vi "Test Write Numerics.vi"(11 "TwinCAT ADS in":refnum<class "TwinCAT ADS.lvclass">) -> (3 "TwinCAT ADS out":refnum<class "TwinCAT ADS.lvclass">)   [LabVIEW 2018]
uses:
  TwinCAT ADS Class/TwinCAT ADS.lvclass
  e70a270d-43c8-4a10-98cb-cdcae2374215.vi
  06e0a99b-7b81-4ca8-a89e-7945807debb3.vi
  d8425a7c-cb21-4544-a4a3-9ee7345751d4.vi
  60045c97-3d21-4f52-bb28-386babca6960.vi
  96827efc-f82d-4e1c-9c1b-454960b395ec.vi
  7e66dc0a-1568-47cd-9851-5dc7b9fa6012.vi
  58f04dc6-9466-4392-88d8-370a7d168ec8.vi
  7dc634db-efdd-42f4-a4b0-d96c414e946f.vi
  TwinCAT ADS Class/VIs/Data/Read.vi
  <vilib>/addons/_JKI Toolkits/Caraya/classes/Assert/Assert Equal Value and Type_Variant.vi
  <vilib>/addons/_JKI Toolkits/Caraya/classes/Assert/Assert Almost Equal_Float.vi
  <vilib>/addons/_JKI Toolkits/Caraya/classes/Assert/Assert.lvclass
  <vilib>/addons/_JKI Toolkits/Caraya/classes/Test/Test.lvclass
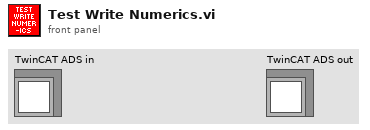
[diagram p1: front panel]
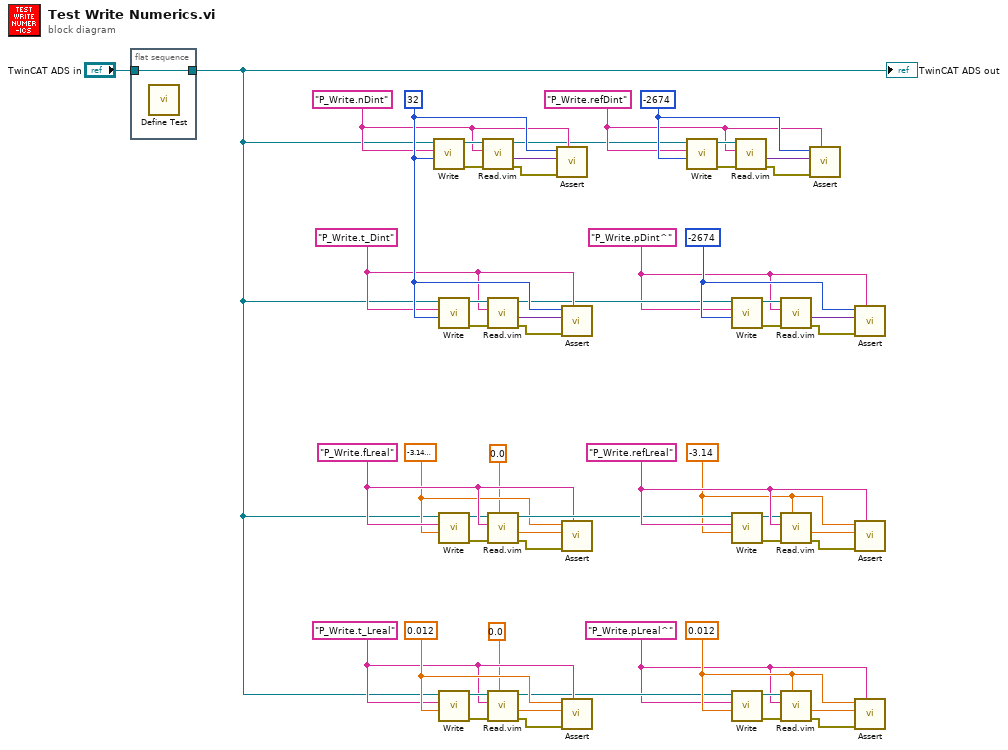
[diagram p0: block diagram]
diagram:
  w14 = 0.012
  w16 = 0.012 ("Value")
  w4 = "P_Write.pLreal^" ("Symbol Name")
  w10 = "P_Write.t_Lreal" ("Symbol Name")
  w19 = -3.140000104904175
  w17 = -3.14 ("Value")
  w29 = "P_Write.refLreal" ("Symbol Name")
  w23 = "P_Write.fLreal" ("Symbol Name")
  w32 = -2674 ("Value")
  w30 = "P_Write.pDint^" ("Symbol Name")
  w39 = -2674 ("Value")
  w38 = "P_Write.refDint" ("Symbol Name")
  w44 = "P_Write.t_Dint" ("Symbol Name")
  w46 = 32 ("Value")
  w45 = "P_Write.nDint" ("Symbol Name")
  n1 = flat-sequence {
    tunnel: "TwinCAT ADS in" -> [w56]
    tunnel: [w56] -> w3
    frame #0 {
      n2 = call <vilib>:"Define Test.vi"() -> ()  [unwired: 10 in, 2 out]
    }
  }
  n3 = call "Write.vi"("Value"=w46, "Symbol Name"=w45, "TwinCAT ADS in"=w3) -> ("error out"=w53:errorcluster, "TwinCAT ADS out"=w54:refnum<class "TwinCAT ADS.lvclass">)  [unwired: 7 in]
  n4 = call "Write.vi"("Value"=w46, "Symbol Name"=w44, "TwinCAT ADS in"=w3) -> ("error out"=w48:errorcluster, "TwinCAT ADS out"=w47:refnum<class "TwinCAT ADS.lvclass">)  [unwired: 7 in]
  n5 = call "Write.vi"("Value"=w19, "Symbol Name"=w23, "TwinCAT ADS in"=w3) -> ("error out"=w21:errorcluster, "TwinCAT ADS out"=w22:refnum<class "TwinCAT ADS.lvclass">)  [unwired: 7 in]
  n6 = call "Write.vi"("Value"=w14, "Symbol Name"=w10, "TwinCAT ADS in"=w3) -> ("error out"=w12:errorcluster, "TwinCAT ADS out"=w11:refnum<class "TwinCAT ADS.lvclass">)  [unwired: 7 in]
  n7 = call "Read.vim"("error in (no error)"=w53, "Symbol Name"=w45, "TwinCAT ADS in"=w54) -> ("error out"=w52:errorcluster, "Value"=w51:variant, "TwinCAT ADS out"=w37:refnum<class "TwinCAT ADS.lvclass">)  [unwired: 6 in]
  n8 = call "Read.vim"("error in (no error)"=w48, "Symbol Name"=w44, "TwinCAT ADS in"=w47) -> ("error out"=w49:errorcluster, "Value"=w50:variant, "TwinCAT ADS out"=w31:refnum<class "TwinCAT ADS.lvclass">)  [unwired: 6 in]
  n9 = call "Read.vim"("Type"=0.0, "error in (no error)"=w21, "Symbol Name"=w23, "TwinCAT ADS in"=w22) -> ("error out"=w20:errorcluster, "Value"=w18:dbl, "TwinCAT ADS out"=w28:refnum<class "TwinCAT ADS.lvclass">)  [unwired: 5 in]
  n10 = call "Read.vim"("Type"=0.0, "error in (no error)"=w12, "Symbol Name"=w10, "TwinCAT ADS in"=w11) -> ("error out"=w13:errorcluster, "Value"=w15:dbl, "TwinCAT ADS out"=w5:refnum<class "TwinCAT ADS.lvclass">)  [unwired: 5 in]
  n11 = call-poly <vilib>:"Assert.vi"("Label"=w45, "error in (no error)"=w52, "Y"=w51, "X"=w46) -> ()  [unwired: 6 in, 2 out]
  n12 = call-poly <vilib>:"Assert.vi"("Label"=w44, "error in (no error)"=w49, "Y"=w50, "X"=w46) -> ()  [unwired: 6 in, 2 out]
  n13 = call-poly <vilib>:"Assert.vi"("Label"=w23, "error in (no error)"=w20, "Y"=w18, "X"=w19) -> ()  [unwired: 6 in, 2 out]
  n14 = call-poly <vilib>:"Assert.vi"("Label"=w10, "error in (no error)"=w13, "Y"=w15, "X"=w14) -> ()  [unwired: 6 in, 2 out]
  n15 = call "Write.vi"("Value"=w39, "Symbol Name"=w38, "TwinCAT ADS in"=w37) -> ("error out"=w42:errorcluster, "TwinCAT ADS out"=w43:refnum<class "TwinCAT ADS.lvclass">)  [unwired: 7 in]
  n16 = call "Write.vi"("Value"=w32, "Symbol Name"=w30, "TwinCAT ADS in"=w31) -> ("error out"=w35:errorcluster, "TwinCAT ADS out"=w36:refnum<class "TwinCAT ADS.lvclass">)  [unwired: 7 in]
  n17 = call "Write.vi"("Value"=w17, "Symbol Name"=w29, "TwinCAT ADS in"=w28) -> ("error out"=w25:errorcluster, "TwinCAT ADS out"=w24:refnum<class "TwinCAT ADS.lvclass">)  [unwired: 7 in]
  n18 = call "Write.vi"("Value"=w16, "Symbol Name"=w4, "TwinCAT ADS in"=w5) -> ("error out"=w8:errorcluster, "TwinCAT ADS out"=w9:refnum<class "TwinCAT ADS.lvclass">)  [unwired: 7 in]
  n19 = call "Read.vim"("error in (no error)"=w42, "Symbol Name"=w38, "TwinCAT ADS in"=w43) -> ("error out"=w41:errorcluster, "Value"=w40:variant)  [unwired: 6 in, 1 out]
  n20 = call "Read.vim"("error in (no error)"=w35, "Symbol Name"=w30, "TwinCAT ADS in"=w36) -> ("error out"=w34:errorcluster, "Value"=w33:variant)  [unwired: 6 in, 1 out]
  n21 = call "Read.vim"("Type"=w17, "error in (no error)"=w25, "Symbol Name"=w29, "TwinCAT ADS in"=w24) -> ("error out"=w26:errorcluster, "Value"=w27:dbl)  [unwired: 5 in, 1 out]
  n22 = call "Read.vim"("Type"=w16, "error in (no error)"=w8, "Symbol Name"=w4, "TwinCAT ADS in"=w9) -> ("error out"=w7:errorcluster, "Value"=w6:dbl)  [unwired: 5 in, 1 out]
  n23 = call-poly <vilib>:"Assert.vi"("Label"=w38, "error in (no error)"=w41, "Y"=w40, "X"=w39) -> ()  [unwired: 6 in, 2 out]
  n24 = call-poly <vilib>:"Assert.vi"("Label"=w30, "error in (no error)"=w34, "Y"=w33, "X"=w32) -> ()  [unwired: 6 in, 2 out]
  n25 = call-poly <vilib>:"Assert.vi"("Label"=w29, "error in (no error)"=w26, "Y"=w27, "X"=w17) -> ()  [unwired: 6 in, 2 out]
  n26 = call-poly <vilib>:"Assert.vi"("Label"=w4, "error in (no error)"=w7, "Y"=w6, "X"=w16) -> ()  [unwired: 6 in, 2 out]
  "TwinCAT ADS out" <- w3
